vi "All Challenges.vi"(8 "error in (no error)":errorcluster, 11 "Challenge DB in":refnum<class "Challenge DB.lvclass">) -> (0 "error out":errorcluster, 2 "Challenges":refnum<class "Challenge.lvclass">[](array[class]), 3 "Challenge DB out":refnum<class "Challenge DB.lvclass">)   [LabVIEW 2020, in "Summer of LabVIEW.lvlib" / "Challenge DB.lvclass"]
uses:
  Challenge DB.lvclass
  Challenge DB.lvclass/Challenge DB.ctl
  Challenge/Challenge.lvclass
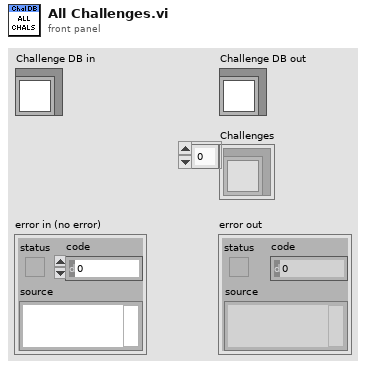
[diagram p1: front panel]
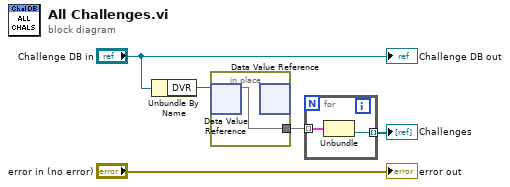
[diagram p0: block diagram]
diagram:
  n1 = Unbundle By Name("Challenge DB in") -> ("DVR"=w4:refnum<data-value>)
  n2 = in-place {
    in-place-border: [w6] -> w2
    n3 = in-place-dvr #1(w4) -> (w6:map{i64, refnum<class "Challenge.lvclass">})  [unwired: 1 out]
    n4 = in-place-dvr #1() -> ()  [unwired: 1 in, 2 out]
  }
  n5 = for {
    tunnel: w2 -> [w8] mode=indexing
    tunnel: [w7] -> w1 mode=indexing
    n6 = Unbundle(w8) -> ("SOL:Challenge.lvclass"=w7:refnum<class "Challenge.lvclass">)  [unwired: 1 out]
  }
  "Challenges" <- w1
  "error out" <- "error in (no error)"
  "Challenge DB out" <- "Challenge DB in"
